vi "Instrument Update Table for Spartan 5.0.vi"(8 "error in (no error)":errorcluster, 11 "Connection Refnum":T1) -> (0 "error out":errorcluster, 3 "Connection Refnum":T1)   [LabVIEW 2011]
uses:
  SI.LIB/ODBC/SQL Controls/Connection Refnum.ctl
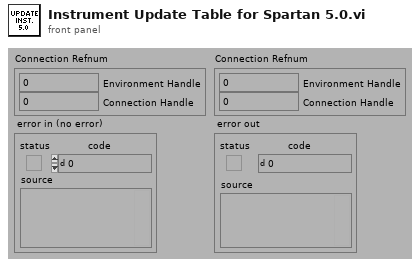
[diagram p1: front panel]
types:
  T1 = typedef "Connection Refnum.ctl" = cluster{"Environment Handle":i32, "Connection Handle":i32}
  T2 = typedef "Statement Refnum.ctl" = cluster{"Statement Handle":i32, "Parameter Number":u16}
  T3 = typedef "Association Record.ctl" = cluster{"ixAssociation":i32, "iStation":i32, "iInstrument":i32}
  T4 = typedef "Instrument Record.ctl" = cluster{"ixInstrument":i32, "sxInstrumentId":string, "sDriverId":string, "sDriverType":string, "sSerialNumber":string, "tLastCalibration":timestamp, "tCalibrationDue":timestamp, "sConfiguration":string}
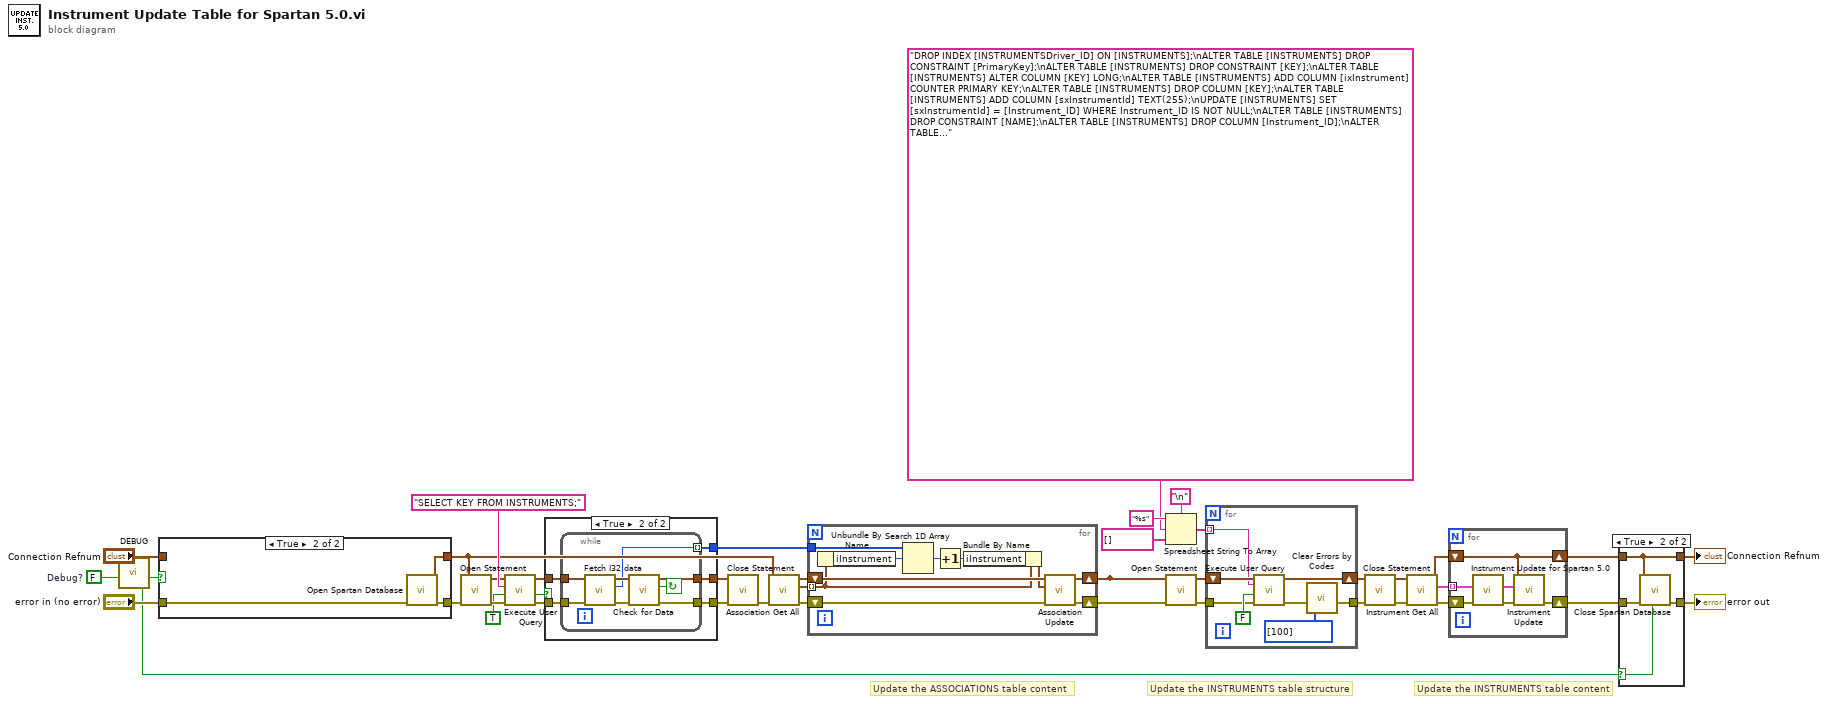
[diagram p0: block diagram]
diagram:
  w27 = FALSE  # Debug?
  # "Update the ASSOCIATIONS table content"
  # "Update the INSTRUMENTS table content"
  # "Update the INSTRUMENTS table structure"
  n1 = call "DEBUG.vi"("Dev DEBUG? (f)"=w27) -> ("DEBUG?"=w26:bool)  [unwired: 1 in, 5 out]
  n2 = case shown="True" w26 {
    tunnel: "Connection Refnum" -> [w41 _]
    tunnel: "error in (no error)" -> [w40 w44]
    tunnel: [w40 w43] -> w5
    tunnel: [w41 w42] -> w3
    frame False {
    }
    frame True {
      n3 = call "Open Spartan Database.vi"("error in (no error)"=w44) -> ("error out"=w43:errorcluster, "Connection Refnum"=w42:T1)  [unwired: 2 in, 7 out]
    }
  }
  n4 = call "Open Statement.vi"("error in (no error)"=w5, "Connection Refnum"=w3) -> ("error out"=w7:errorcluster, "Statement Refnum"=w6:T2)  [unwired: 4 out]
  n5 = call "Execute User Query.vi"("error in (no error)"=w7, "Return Data? (f)"=TRUE, "User Query"="SELECT KEY FROM INSTRUMENTS;", "Statement Refnum"=w6) -> ("error out"=w17:errorcluster, "Data Present?"=w18:bool, "Statement Refnum"=w16:T2)  [unwired: 1 out]
  n6 = case shown="True" w18 {
    tunnel: w17 -> [w45 w49]
    tunnel: w16 -> [w46 w50]
    tunnel: [w45 w48] -> w15
    tunnel: [w46 w47] -> w14
    tunnel: [_ w51] -> w9
    frame False {
    }
    frame True {
      n7 = while {
        tunnel: [w56] -> w51 mode=indexing
        tunnel: w50 -> [w55]
        tunnel: w49 -> [w54]
        tunnel: [w53] -> w48
        tunnel: [w52] -> w47
        stop <- w57 continue-if-true
        n8 = call "Fetch I32 data.vi"("error in (no error)"=w54, "Statement Refnum"=w55) -> ("error out"=w59:errorcluster, "Data"=w56:i32, "Statement Refnum"=w58:T2)  [unwired: 3 out]
        n9 = call "Check for Data.vi"("error in (no error)"=w59, "Statement Refnum"=w58) -> ("error out"=w53:errorcluster, "Data Present?"=w57:bool, "Statement Refnum"=w52:T2)  [unwired: 3 out]
      }
    }
  }
  n10 = call "Close Statement.vi"("error in (no error)"=w15, "Statement Refnum"=w14) -> ("error out"=w13:errorcluster)  [unwired: 5 out]
  n11 = call "Association Get All.vi"("error in (no error)"=w13, "Connection Refnum"=w3) -> ("error out"=w12:errorcluster, "Associations"=w10:T3[], "Connection Refnum"=w11:T1)  [unwired: 7 out]
  n12 = for {
    shift-right: [w69] -> w4
    shift-left: w12 -> [w67]
    tunnel: w10 -> [w63] mode=indexing
    shift-right: [w68] -> w8
    shift-left: w11 -> [w66]
    tunnel: w9 -> [w65]
    n13 = Unbundle By Name(w63) -> ("iInstrument"=w64:i32)
    n14 = Search 1D Array(1D array=w65, element=w64) -> (index of element=w60:i32)  [unwired: 1 out]
    n15 = Increment(x=w60) -> (x+1=w61:i32)
    n16 = Bundle By Name(cluster=w63, "iInstrument"=w61) -> (w62:T3)
    n17 = call "Association Update.vi"("error in (no error)"=w67, "Association Record (empty)"=w62, "Connection Refnum"=w66) -> ("error out"=w69:errorcluster, "Connection Refnum"=w68:T1)  [unwired: 7 out]
  }
  n18 = Spreadsheet String To Array(delimiter (Tab)="\n", format string="%s", spreadsheet string="DROP INDEX [INSTRUMENTSDriver_ID] ON [INSTRUMENTS];\nALTER TABLE [INSTRUMENTS] DROP CONSTRAINT [PrimaryKey];\nALTER TABLE [INSTRUMENTS] DROP CONSTRAINT [KEY];\nALTER TABLE [INSTRUMENTS] ALTER COLUMN [KEY] LONG;\nALTER TABLE [INSTRUMENTS] ADD COLUMN [ixInstrument] COUNTER PRIMARY KEY;\nALTER TABLE [INSTRUMENTS] DROP COLUMN [KEY];\nALTER TABLE [INSTRUMENTS] ADD COLUMN [sxInstrumentId] TEXT(255);\nUPDATE [INSTRUMENTS] SET [sxInstrumentId] = [Instrument_ID] WHERE Instrument_ID IS NOT NULL;\nALTER TABLE [INSTRUMENTS] DROP CONSTRAINT [NAME];\nALTER TABLE [INSTRUMENTS] DROP COLUMN [Instrument_ID];\nALTER TABLE [INSTRUMENTS] ADD COLUMN [sDriverId] TEXT(255);\nUPDATE [INSTRUMENTS] SET [sDriverId] = [Driver_ID];\nALTER TABLE [INSTRUMENTS] DROP COLUMN [Driver_ID];\nALTER TABLE [INSTRUMENTS] ADD COLUMN [sDriverType] TEXT(255);\nUPDATE [INSTRUMENTS] SET [sDriverType] = [DriverType];\nALTER TABLE [INSTRUMENTS] DROP COLUMN [DriverType];\nALTER TABLE [INSTRUMENTS] ADD COLUMN [sSerialNumber] TEXT(255);\nUPDATE [INSTRUMENTS] SET [sSerialNumber] = [Serial_Number];\nALTER TABLE [INSTRUMENTS] DROP CONSTRAINT [Serial_Number];\nALTER TABLE [INSTRUMENTS] DROP COLUMN [Serial_Number];\nALTER TABLE [INSTRUMENTS] ADD COLUMN [sTemp] TEXT(255);\nUPDATE [INSTRUMENTS] SET [sTemp] = [Last_Cal];\nALTER TABLE [INSTRUMENTS] DROP COLUMN [Last_Cal];\nUPDATE [INSTRUMENTS] SET [sDriverType] = [sDriverType]+'-'+[sTemp];\nUPDATE [INSTRUMENTS] SET [sTemp] = [Cal_Due];\nALTER TABLE [INSTRUMENTS] DROP COLUMN [Cal_Due];\nUPDATE [INSTRUMENTS] SET [sDriverType] = [sDriverType]+'-'+[sTemp];\nALTER TABLE [INSTRUMENTS] DROP COLUMN [sTemp];\nALTER TABLE [INSTRUMENTS] ADD COLUMN [tLastCalibration] DATE;\nALTER TABLE [INSTRUMENTS] ADD COLUMN [tCalibrationDue] DATE;\nALTER TABLE [INSTRUMENTS] ADD COLUMN [sConfiguration] TEXT(255);\nUPDATE [INSTRUMENTS] SET [sConfiguration] = [Configuration];\nALTER TABLE [INSTRUMENTS] DROP COLUMN [Configuration];" ("User Query"), array type (2D Dbl)=string[] []) -> (array=w38:string[])
  n19 = call "Open Statement.vi"("error in (no error)"=w4, "Connection Refnum"=w8) -> ("error out"=w35:errorcluster, "Statement Refnum"=w34:T2)  [unwired: 4 out]
  n20 = for {
    tunnel: w38 -> [w76] mode=indexing
    shift-right: [w73] -> w32
    shift-left: w34 -> [w75]
    tunnel: w35 -> [w74]
    tunnel: [w70] -> w33
    n21 = call "Execute User Query.vi"("error in (no error)"=w74, "Return Data? (f)"=FALSE, "User Query"=w76, "Statement Refnum"=w75) -> ("error out"=w71:errorcluster, "Statement Refnum"=w73:T2)  [unwired: 2 out]
    n22 = call "Clear Errors by Codes.vi"("Error Codes\nto Clear (Empty)"=i32[] [100] ("Error Codes\nto Clear (Empty)"), "error in (no error)"=w71) -> ("error out"=w70:errorcluster)  [unwired: 5 out]
  }
  n23 = call "Close Statement.vi"("error in (no error)"=w33, "Statement Refnum"=w32) -> ("error out"=w22:errorcluster)  [unwired: 5 out]
  n24 = call "Instrument Get All.vi"("error in (no error)"=w22, "Connection Refnum"=w8) -> ("error out"=w23:errorcluster, "Instruments"=w25:T4[], "Connection Refnum"=w24:T1)  [unwired: 2 in, 5 out]
  n25 = for {
    shift-right: [w83] -> w21
    shift-left: w23 -> [w81]
    shift-right: [w82] -> w20
    shift-left: w24 -> [w82]
    tunnel: w25 -> [w78] mode=indexing
    n26 = call "Instrument Update for Spartan 5.0.vi"("error in (no error)"=w81, "Old Instrument Record"=w78) -> ("error out"=w80:errorcluster, "New Instrument Record"=w79:T4)  [unwired: 8 out]
    n27 = call "Instrument Update.vi"("error in (no error)"=w80, "Instrument Record"=w79, "Connection Refnum"=w82) -> ("error out"=w83:errorcluster)  [unwired: 8 out]
  }
  n28 = case shown="True" w26 {
    selector: w26 -> [_ w87]
    tunnel: w21 -> [w85 w89]
    tunnel: w20 -> [w84 w86]
    tunnel: [w84 w86] -> w31
    tunnel: [w85 w88] -> w30
    frame False {
    }
    frame True {
      n29 = call "Close Spartan Database.vi"("Force Close? (f)"=w87, "error in (no error)"=w89, "Connection Refnum"=w86) -> ("error out"=w88:errorcluster)  [unwired: 2 in, 6 out]
    }
  }
  "error out" <- w30
  "Connection Refnum" <- w31
